vi "Write Create Room Service Request Msg.vi"(10 "Room Service Manager UI.lvlib:Create Room Service Request Msg.lvclass":refnum<class "Create Room Service Request Msg.lvclass">, 11 "Room Service Manager UI in":refnum<class "Room Service Manager UI.lvclass">) -> (3 "Room Service Manager UI out":refnum<class "Room Service Manager UI.lvclass">)   [LabVIEW 2023, in "Room Service Manager UI.lvlib" / "Room Service Manager UI.lvclass"]
uses:
  Room Service Manager UI.lvclass
  Room Service Manager UI Messages/Create Room Service Request Msg/Create Room Service Request Msg.lvclass
  Room Service Manager UI.lvclass/Room Service Manager UI.ctl
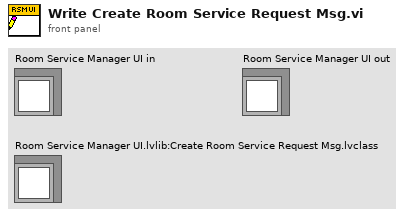
[diagram p1: front panel]
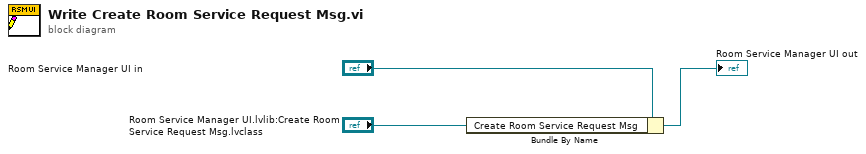
[diagram p0: block diagram]
diagram:
  n1 = Bundle By Name(cluster="Room Service Manager UI in", "Create Room Service Request Msg"="Room Service Manager UI.lvlib:Create Room Service Request Msg.lvclass") -> (→"Room Service Manager UI out":refnum<class "Room Service Manager UI.lvclass">)
